vi "Count Groups.vi"(8 "error in":errorcluster, 10 "regular expression":string="^s", 11 "tdms file":refnum<k34>) -> (0 "error out":errorcluster, 1 "group names":string[](array[string]), 2 "Count":i32, 3 "tdms file out":refnum<k34>)   [LabVIEW 2021]
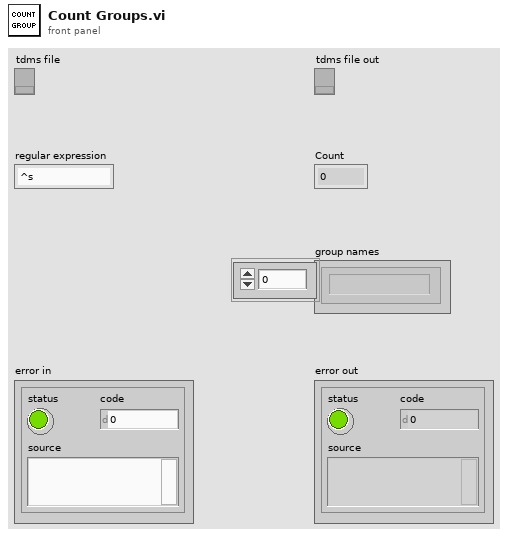
[diagram p1: front panel]
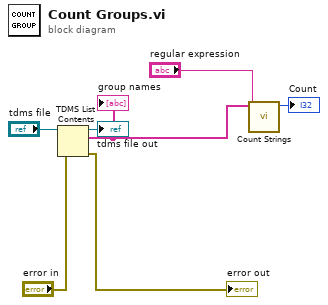
[diagram p0: block diagram]
diagram:
  n1 = TDMS List Contents(4:"error in", 7:"tdms file") -> (0:→"error out":errorcluster, 2:w3:string[], 3:→"tdms file out":refnum<k34>)  [unwired: 1 in, 1 out]
  "group names" <- w3
  n2 = call "Count Strings.vi"("regular expression"="regular expression", "Array - String"=w3) -> ("Count"=→"Count":i32)  [unwired: 9 in]
